vi "DATA_CONV.vi"(0 "phasors in":csg[](array[numeric]), 1 "format":u16, 5 "freq in":sgl, 9 "dfreq in":sgl, 11 "analogs in":sgl[](array[numeric]), 12 "phasor units":u32[](array[numeric]), 13 "nominal frequency":enum16{"50 Hz", "60 Hz"}(ring)) -> (2 "analog out of range":bool, 3 "freq out of range":bool, 4 "phasor byte array":u8[](array[numeric]), 6 "freq byte array":u8[](array[numeric]), 8 "df/dt out of range":bool, 10 "dfreq byte array":u8[](array[numeric]), 14 "phasor out of range":bool, 15 "analogs byte array":u8[](array[numeric]))   [LabVIEW 2013]
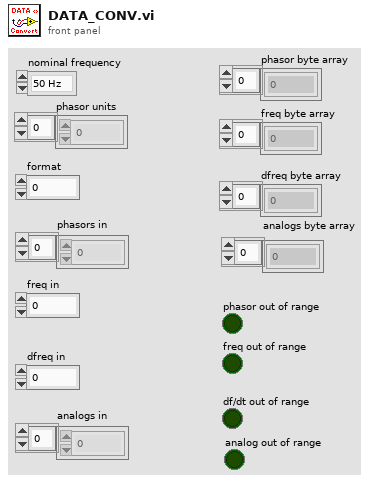
[diagram p1: front panel]
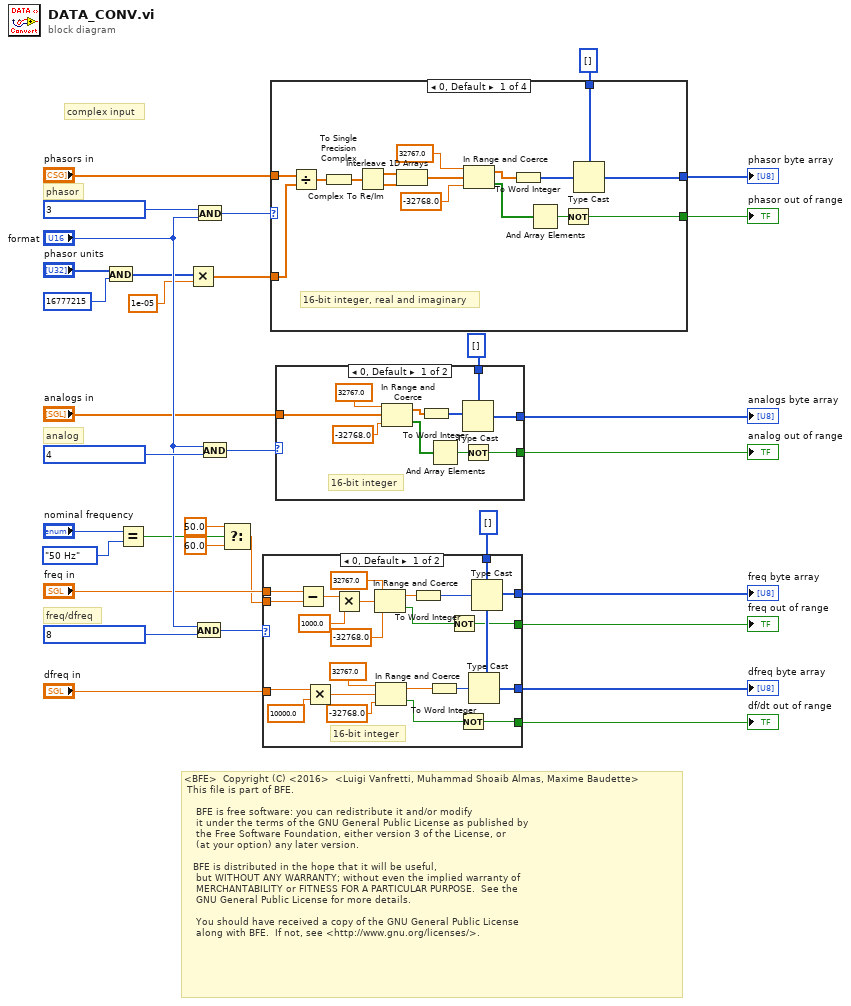
[diagram p0: block diagram]
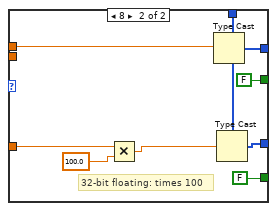
[diagram p2: hidden frame]
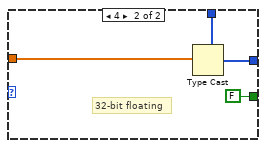
[diagram p3: hidden frame]
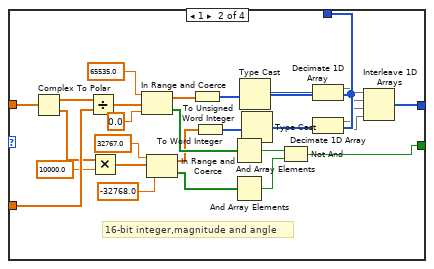
[diagram p4: hidden frame]
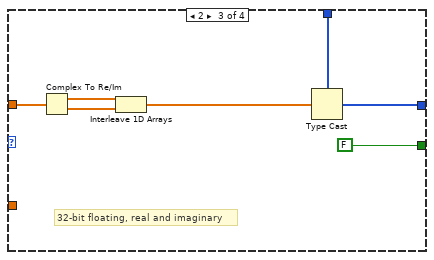
[diagram p5: hidden frame]
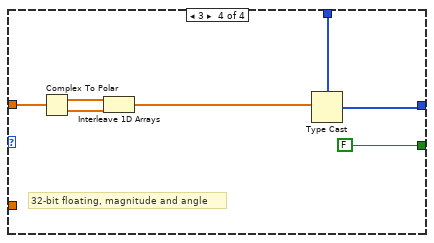
[diagram p6: hidden frame]
diagram:
  # "<BFE>  Copyright (C) <2016>  <Luigi Vanfretti, Muhammad Shoaib Almas, Maxime Baudette>\n This file is part of BFE.\n\n    BFE is free software: you can redistribute it and/or modify\n    it under the terms of the GNU General Public License as published by\n    the Free Software Foundation, either version 3 of the License, or\n    (at your option) any later version.\n\n   BFE is distributed in the hope that it will be useful,\n    but WITHOUT ANY WARRANTY; without even the implied warranty of\n    MERCHANTABILITY or FITNESS FOR A PARTICULAR PURPOSE.  See the\n    GNU General Public License for more details.\n\n    You should have received a copy of the GNU General Public License\n    along with BFE.  If not, see <http://www.gnu.org/licenses/>."
  # "complex input"
  # "freq/dfreq"
  # "analog"
  # "phasor"
  n1 = And(x="phasor units", y=u32 16777215) -> (x .and. y?=w13:u32[])
  n2 = Equal?(x="nominal frequency", y=enum16{"50 Hz", "60 Hz"}."50 Hz" ("nominal frequency 2")) -> (x = y?=w7:bool)
  n3 = Multiply(x=w13, y=1e-05) -> (x*y=w11:dbl[])
  n4 = And(x="format", y=u16 8 ("x")) -> (x .and. y?=w24:u16)
  n5 = And(x=u16 3, y="format") -> (x .and. y?=w29:u16)
  n6 = And(x="format", y=u16 4 ("x")) -> (x .and. y?=w25:u16)
  n7 = Select(t=50.0, s=w7, f=60.0) -> (s? t:f=w4:dbl)
  n8 = case shown="0, Default" w24 {
    tunnel: "freq in" -> [w52 w62]
    tunnel: "dfreq in" -> [w40 w58]
    tunnel: u8[] [] ("appended array") -> [w55 w64]
    tunnel: [w56 w65] -> w17
    tunnel: [w53 w63] -> w16
    tunnel: w4 -> [w51 _]
    tunnel: [w36 FALSE] -> w3
    tunnel: [w35 FALSE] -> w2
    frame 0, Default {
      # "16-bit integer"
      n9 = Subtract(x=w52, y=w51) -> (x-y=w50:dbl)
      n10 = Multiply(x=w40, y=sgl 10000.0) -> (x*y=w38:sgl)
      n11 = Multiply(x=w50, y=1000.0) -> (x*y=w48:dbl)
      n12 = In Range and Coerce(upper limit=32767.0 ("y"), x=w48, lower limit=-32768.0 ("y")) -> (coerced(x)=w45:dbl, In Range?=w37:bool)
      n13 = In Range and Coerce(upper limit=sgl 32767.0 ("y"), x=w38, lower limit=sgl -32768.0 ("y")) -> (coerced(x)=w41:sgl, In Range?=w34:bool)
      n14 = To Word Integer(number=w45) -> (16bit integer=w44:i16)
      n15 = To Word Integer(number=w41) -> (16bit integer=w54:i16)
      n16 = Not(x=w37) -> (.not. x?=w36:bool)
      n17 = Not(x=w34) -> (.not. x?=w35:bool)
      n18 = Type Cast(type=w55, x=w54) -> (*(type *) &x=w53:u8[])
      n19 = Type Cast(type=w55, x=w44) -> (*(type *) &x=w56:u8[])
    }
    frame 8 {
      # "32-bit floating: times 100"
      n20 = Multiply(x=w58, y=sgl 100.0) -> (x*y=w57:sgl)
      n21 = Type Cast(type=w64, x=w62) -> (*(type *) &x=w65:u8[])
      n22 = Type Cast(type=w64, x=w57) -> (*(type *) &x=w63:u8[])
    }
  }
  "freq byte array" <- w17
  "dfreq byte array" <- w16
  "freq out of range" <- w3
  "df/dt out of range" <- w2
  n23 = case shown="0, Default" w29 {
    tunnel: "phasors in" -> [w76 w109 w116 w123]
    tunnel: u8[] [] ("appended array") -> [w81 w90 w112 w119]
    tunnel: [w80 w83 w111 w118] -> w26
    tunnel: w11 -> [w75 w107 _ _]
    tunnel: [w66 w82 FALSE FALSE] -> w10
    frame 0, Default {
      # "16-bit integer, real and imaginary"
      n24 = Divide(x=w76, y=w75) -> (x/y=w74:cdb[])
      n25 = To Single Precision Complex(1:w74) -> (0:w73:csg[])
      n26 = Complex To Re/Im(x + iy=w73) -> (x=w79:sgl[], y=w78:sgl[])
      n27 = Interleave 1D Arrays(w79, w78) -> (w72:sgl[])
      n28 = In Range and Coerce(upper limit=sgl 32767.0, x=w72, lower limit=sgl -32768.0) -> (coerced(x)=w69:sgl[], In Range?=w68:bool[])
      n29 = To Word Integer(number=w69) -> (16bit integer=w77:i16[])
      n30 = And Array Elements(Boolean array=w68) -> (logical AND=w67:bool)
      n31 = Not(x=w67) -> (.not. x?=w66:bool)
      n32 = Type Cast(type=w81, x=w77) -> (*(type *) &x=w80:u8[])
    }
    frame 1 {
      # "16-bit integer,magnitude and angle"
      n33 = Complex To Polar(r * e^(i*theta)=w109) -> (r=w108:sgl[], theta=w106:sgl[])
      n34 = Divide(x=w108, y=w107) -> (x/y=w104:dbl[])
      n35 = Multiply(x=w106, y=sgl 10000.0) -> (x*y=w101:sgl[])
      n36 = In Range and Coerce(upper limit=65535.0, x=w104, lower limit=0.0) -> (coerced(x)=w95:dbl[], In Range?=w98:bool[])
      n37 = In Range and Coerce(upper limit=sgl 32767.0, x=w101, lower limit=sgl -32768.0) -> (coerced(x)=w94:sgl[], In Range?=w92:bool[])
      n38 = To Unsigned Word Integer(number=w95) -> (unsigned 16bit integer=w93:u16[])
      n39 = To Word Integer(number=w94) -> (16bit integer=w91:i16[])
      n40 = And Array Elements(Boolean array=w98) -> (logical AND=w97:bool)
      n41 = And Array Elements(Boolean array=w92) -> (logical AND=w96:bool)
      n42 = Type Cast(type=w90, x=w93) -> (*(type *) &x=w89:u8[])
      n43 = Type Cast(type=w90, x=w91) -> (*(type *) &x=w88:u8[])
      n44 = Not And(1:w96, 2:w97) -> (0:w82:bool)
      n45 = Decimate 1D Array(w89) -> (w87:u8[], w86:u8[])
      n46 = Decimate 1D Array(w88) -> (w85:u8[], w84:u8[])
      n47 = Interleave 1D Arrays(w87, w86, w85, w84) -> (w83:u8[])
    }
    frame 2 {
      # "32-bit floating, real and imaginary"
      n48 = Complex To Re/Im(x + iy=w116) -> (x=w115:sgl[], y=w114:sgl[])
      n49 = Interleave 1D Arrays(w115, w114) -> (w113:sgl[])
      n50 = Type Cast(type=w112, x=w113) -> (*(type *) &x=w111:u8[])
    }
    frame 3 {
      # "32-bit floating, magnitude and angle"
      n51 = Complex To Polar(r * e^(i*theta)=w123) -> (r=w122:sgl[], theta=w121:sgl[])
      n52 = Interleave 1D Arrays(w122, w121) -> (w120:sgl[])
      n53 = Type Cast(type=w119, x=w120) -> (*(type *) &x=w118:u8[])
    }
  }
  "phasor byte array" <- w26
  "phasor out of range" <- w10
  n54 = case shown="0, Default" w25 {
    tunnel: "analogs in" -> [w128 w136]
    tunnel: u8[] [] ("appended array") -> [w132 w137]
    tunnel: [w131 w135] -> w21
    tunnel: [w124 FALSE] -> w1
    frame 0, Default {
      # "16-bit integer"
      n55 = In Range and Coerce(upper limit=sgl 32767.0 ("y"), x=w128, lower limit=sgl -32768.0 ("y")) -> (coerced(x)=w127:sgl[], In Range?=w125:bool[])
      n56 = To Word Integer(number=w127) -> (16bit integer=w133:i16[])
      n57 = And Array Elements(Boolean array=w125) -> (logical AND=w126:bool)
      n58 = Type Cast(type=w132, x=w133) -> (*(type *) &x=w131:u8[])
      n59 = Not(x=w126) -> (.not. x?=w124:bool)
    }
    frame 4 {
      # "32-bit floating"
      n60 = Type Cast(type=w137, x=w136) -> (*(type *) &x=w135:u8[])
    }
  }
  "analogs byte array" <- w21
  "analog out of range" <- w1
